vi "signal-test.vi"() -> ()   [LabVIEW 2018]
panel:
  out "Leistung":dynamicdata(graph)
  out "Spannung":dynamicdata(graph)
  out "Strom":dynamicdata(graph)
  in  "Verstärkung Bremsmoment":dbl
  out "Bremsmoment genähert, ungefiltert":dynamicdata(graph)
  in  "stop (F)":bool
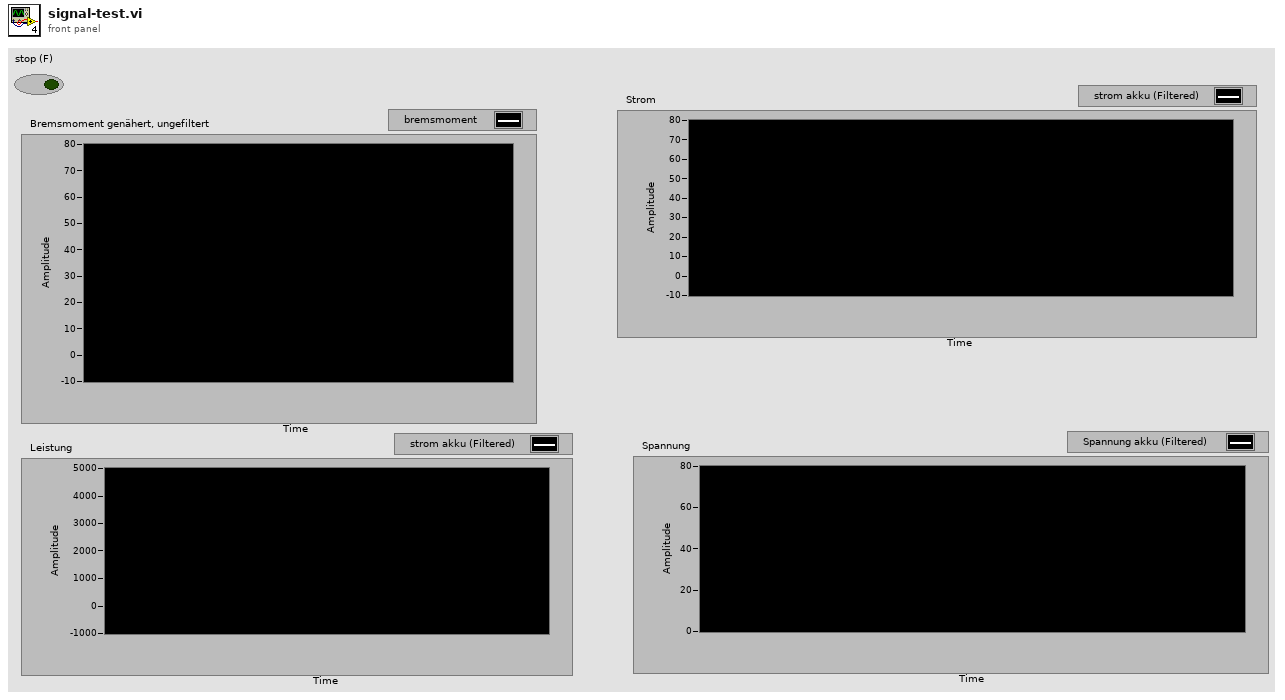
[diagram p1: front panel]
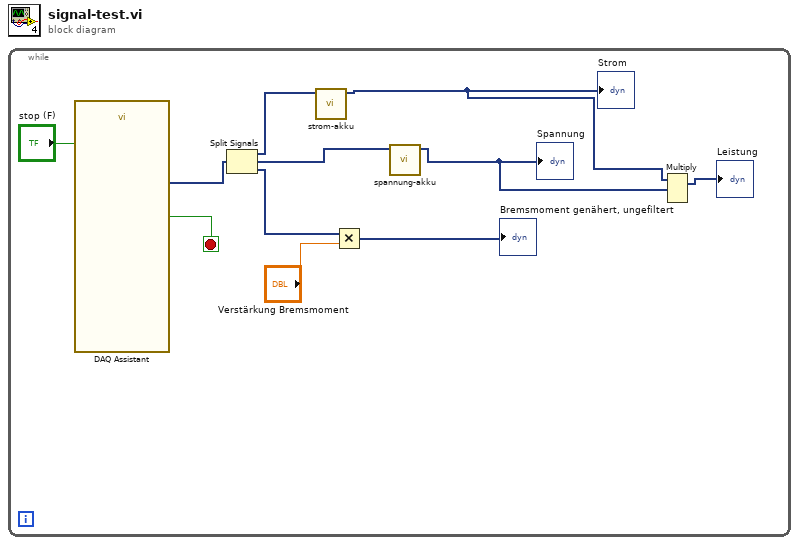
[diagram p0: block diagram]
diagram:
  n1 = while {
    stop <- w10 stop-if-true
    n2 = call "DAQ Assistant"("stop (F)"="stop (F)") -> ("data"=w9:dynamicdata, "stopped"=w10:bool)  [unwired: 15 in, 2 out]
    n3 = Split Signals(w9) -> (w5:dynamicdata, w4:dynamicdata, w8:dynamicdata)  [unwired: 3 in]
    n4 = call "strom-akku.vi"("Dynamic Data"=w5) -> ("Filtered Signal"=w3:dynamicdata)  [unwired: 10 in]
    "Strom" <- w3
    n5 = Multiply(x=w8, y="Verstärkung Bremsmoment") -> (x*y=→"Bremsmoment genähert, ungefiltert":dynamicdata)
    n6 = call "spannung-akku.vi"("Dynamic Data in"=w4) -> ("Dynamic Data out"=w2:dynamicdata)  [unwired: 10 in]
    "Spannung" <- w2
    n7 = Multiply(1:w2, 2:w3) -> (0:→"Leistung":dynamicdata)  [unwired: 1 in, 1 out]
  }
